vi "RunSEQ.vi"(0 "VISA resource name":refnum<visa-resource-name>, 1 "Amp or Ohm?":bool=TRUE, 4 "Ramp + Dwell Time (s)":string, 5 "Sequence Number":string, 6 "Step Number":string, 7 "error in (no error)":errorcluster) -> (14 "Step Status":string, 15 "Peak ARC Current (uA)":dbl, 16 "Test Step Status Description":string, 17 "Measurement Result Unit":string, 18 "Execution Status":string, 19 "Measurement Result (uA or mOhm)":dbl caption="Measurement Result(uA)", 20 "VISA resource name out":refnum<visa-resource-name>, 21 "Elapsed Time (s)":dbl, 22 "Final Test Level (A or V)":dbl, 23 "Peak Breakdown Current (uA)":dbl caption="Peak Breakdown Current(uA)", 24 "Peak Breakdown Current Unit":string, 25 "Error Message":string, 26 "Error Code":i32, 27 "error out":errorcluster)   [LabVIEW 2010, in "VITREK V7X.lvlib"]
doc: "Run a specified sequence."
uses:
  VITREK V7X.lvlib
  Instance           2 14Saved   RunSEQ .vi
  Instance           1 14Saved   RunSEQ .vi
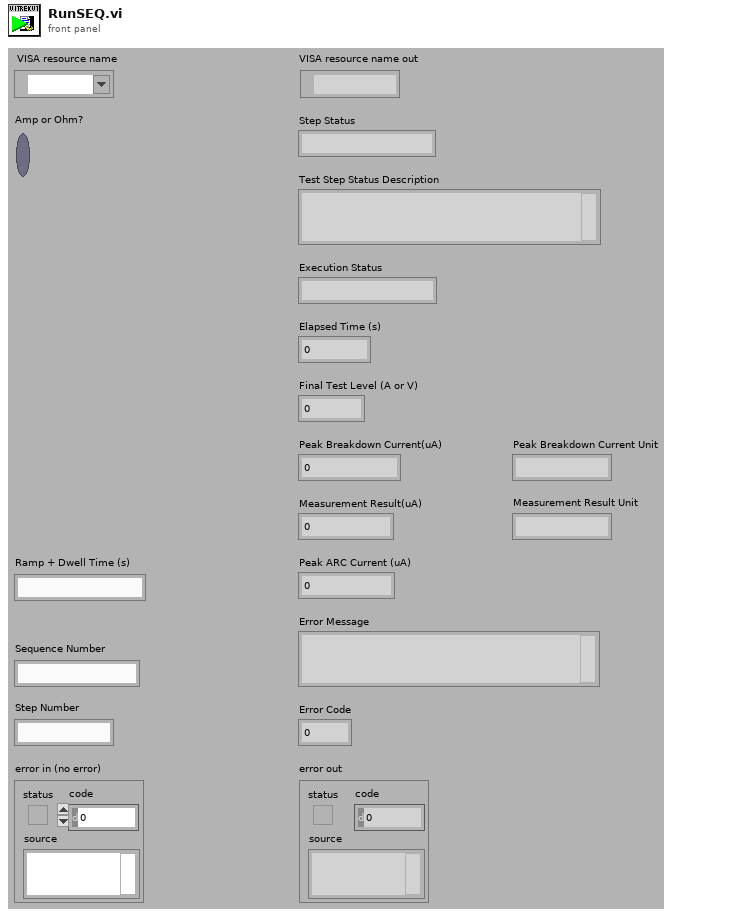
[diagram p1: front panel]
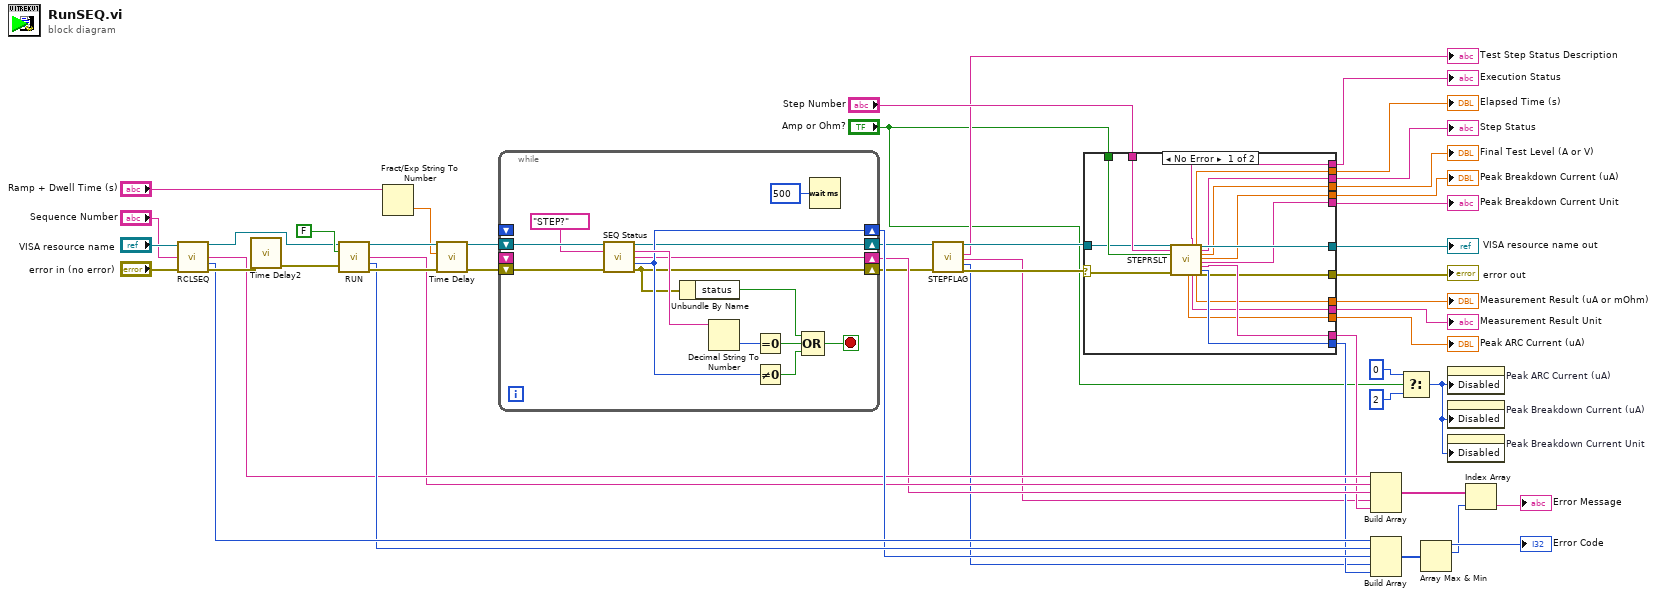
[diagram p0: block diagram]
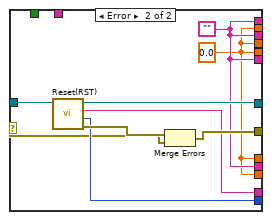
[diagram p2: hidden frame]
diagram:
  n1 = call "RCLSEQ.vi"("VISA resource name"="VISA resource name", "Sequence Number"="Sequence Number", "error in (no error)"="error in (no error)") -> ("VISA resource name out"=w41:refnum<visa-resource-name>, "Error Message"=w32:string, "Error Code"=w35:i32, "error out"=w42:errorcluster)  [unwired: 9 in]
  n2 = call "Time Delay2"("error in (no error)"=w42) -> ("error out"=w5:errorcluster)  [unwired: 10 in]
  n3 = call "RUN.vi"("VISA resource name"=w41, "Run Query"=FALSE, "error in (no error)"=w5) -> ("VISA resource name out"=w39:refnum<visa-resource-name>, "Error Message"=w31:string, "Error Code"=w34:i32, "error out"=w40:errorcluster)  [unwired: 8 in, 1 out]
  n4 = Fract/Exp String To Number(string="Ramp + Dwell Time (s)") -> (number=w36:dbl)  [unwired: 3 in, 1 out]
  n5 = call "Time Delay"("error in (no error)"=w40, "Delay Time (s)"=w36) -> ("error out"=w38:errorcluster)  [unwired: 9 in]
  n6 = while {
    shift-right: [w53] -> w12
    shift-left: w38 -> [w57]
    shift-right: [w56] -> w33
    shift-left: _ -> [_]
    shift-right: [w55] -> w26
    shift-left: _ -> [_]
    shift-right: [w54] -> w9
    shift-left: w39 -> [w62]
    stop <- w50 stop-if-true
    n7 = call "SEQ Status.vi"("VISA resource name"=w62, "Status Selection"="STEP?", "error in (no error)"=w57) -> ("VISA resource name out"=w54:refnum<visa-resource-name>, "Status Output"=w59:string, "Error Message"=w55:string, "Error Code"=w56:i32, "error out"=w53:errorcluster)  [unwired: 8 in]
    n8 = Unbundle By Name(w53) -> ("status"=w49:bool)
    n9 = Decimal String To Number(string=w59) -> (number=w58:i32)  [unwired: 2 in, 1 out]
    n10 = Equal To 0?(x=w58) -> (x = 0?=w51:bool)
    n11 = Not Equal To 0?(x=w56) -> (x != 0?=w52:bool)
    n12 = Compound Arithmetic op=OR(w49, w51, w52) -> (w50:bool)
    n13 = Wait (ms)(milliseconds to wait=u32 500) -> ()  [unwired: 1 out]
  }
  n14 = call "STEPFLAG.vi"("VISA resource name"=w9, "error in (no error)"=w12) -> ("VISA resource name out"=w10:refnum<visa-resource-name>, "Test Step Status Description"=→"Test Step Status Description":string, "Error Message"=w7:string, "Error Code"=w8:i32, "error out"=w11:errorcluster)  [unwired: 12 in, 1 out]
  n15 = case shown="No Error" w11 {
    selector: w11 -> [w64 w82]
    tunnel: w10 -> [w63 w88]
    tunnel: "Step Number" -> [w79 _]
    tunnel: "Amp or Ohm?" -> [w65 _]
    tunnel: [w78 w83] -> w25
    tunnel: [w77 w84] -> w24
    tunnel: [w76 w85] -> w23
    tunnel: [w75 w86] -> w22
    tunnel: [w74 w81] -> w21
    tunnel: [w73 w80] -> w20
    tunnel: [w72 w81] -> w19
    tunnel: [w71 w80] -> w18
    tunnel: [w70 w80] -> w17
    tunnel: [w69 w81] -> w16
    tunnel: [w68 w80] -> w15
    tunnel: [w67 w81] -> w14
    tunnel: [w66 w80] -> w13
    frame No Error {
      n16 = call "STEPRSLT.vi"("VISA resource name"=w63, "Step Number"=w79, "Amp or Ohm?"=w65, "error in (no error)"=w64) -> ("Peak ARC Current (uA)"=w66:dbl, "Execution Status"=w74:string, "Measurement Result Unit"=w67:string, "Elapsed Time (s)"=w73:dbl, "Measurement Result (uA or mOhm)"=w68:dbl, "VISA resource name out"=w76:refnum<visa-resource-name>, "Step Status"=w72:string, "Final Test Level (A or V)"=w71:dbl, "Peak Breakdown Current (uA)"=w70:dbl, "Peak Breakdown Current Unit"=w69:string, "Error Message"=w78:string, "Error Code"=w77:i32, "error out"=w75:errorcluster)  [unwired: 10 in, 1 out]
    }
    frame Error {
      w80 = 0.0 ("Peak Breakdown Current (uA)")
      w81 = ""
      n17 = call "Reset(RST).vi"("VISA resource name"=w88) -> ("error out"=w87:errorcluster, "Error Code"=w84:i32, "Error Message"=w83:string, "VISA resource name out"=w85:refnum<visa-resource-name>)  [unwired: 7 in]
      n18 = Merge Errors(w87, w82) -> (w86:errorcluster)
    }
  }
  "error out" <- w22
  "VISA resource name out" <- w23
  "Execution Status" <- w21
  "Elapsed Time (s)" <- w20
  "Step Status" <- w19
  "Final Test Level (A or V)" <- w18
  "Peak Breakdown Current (uA)" <- w17
  "Peak Breakdown Current Unit" <- w16
  "Measurement Result (uA or mOhm)" <- w15
  "Measurement Result Unit" <- w14
  "Peak ARC Current (uA)" <- w13
  n19 = Build Array(w32, w31, w26, w7, w25) -> (w48:string[])
  n20 = Build Array(w35, w34, w33, w8, w24) -> (w46:i32[])
  n21 = Select(t=0, s="Amp or Ohm?", f=2) -> (s? t:f=w1:i32)
  n22 = Array Max & Min(array=w46) -> (max value=→"Error Code":i32, max index (indices)=w44:i32)  [unwired: 2 out]
  n23 = property on="Peak ARC Current (uA)" class="DigNum (strict)"("Disabled"=w1) -> ()  [unwired: 2 in, 2 out]
  n24 = property on="Peak Breakdown Current (uA)" class="DigNum (strict)"("Disabled"=w1) -> ()  [unwired: 2 in, 2 out]
  n25 = property on="Peak Breakdown Current Unit" class="Str"("Disabled"=w1) -> ()  [unwired: 2 in, 2 out]
  n26 = Index Array(array=w48, index=w44) -> (element=→"Error Message":string)
